vi "Take Composite Image.vi"(7 "Quality":enum16{"perfect", "medium", "low"}(ring), 8 "error in":errorcluster, 9 "Image Name":string="composite image", 10 "Points":refnum<class "Vec3d Class.lvclass">[](array[class]), 11 "CameraTool in":refnum<class "CameraTool Class.lvclass">) -> (0 "error out":errorcluster, 2 "Physical Image":T1, 3 "CameraTool out":refnum<class "CameraTool Class.lvclass">)   [LabVIEW 2011, in "CameraTool Class.lvclass"]
uses:
  CameraTool Class.lvclass
  Vec3d Class/Vec3d Class.lvclass
  Utils/Type Definitions/Physical Image.ctl
  <vilib>/vision/Image Controls.llb/IMAQ Image.ctl
  Config Manager Class/Type Definitions/Camera Enum.ctl
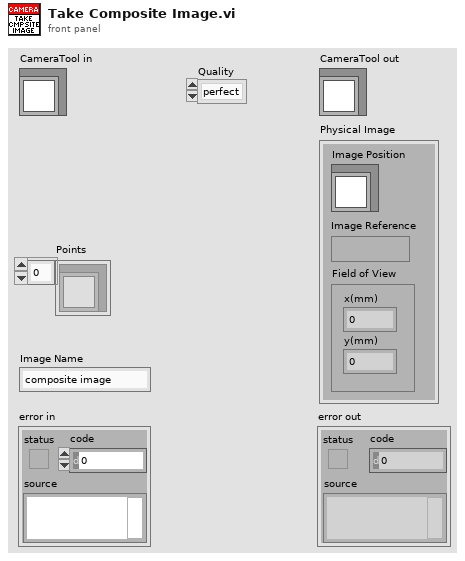
[diagram p1: front panel]
types:
  T1 = typedef "Physical Image.ctl" = cluster{"Image Position":refnum<class "Vec3d Class.lvclass">, "Image Reference":T2, "Field of View":cluster{"x(mm)":dbl, "y(mm)":dbl}}
  T2 = typedef "IMAQ Image.ctl" = refnum<image>
  T3 = typedef "Camera Enum.ctl" = enum16{"GANTRY HEAD", "NEEDLE CALIBRATION X", "NEEDLE CALIBRATION Y"}
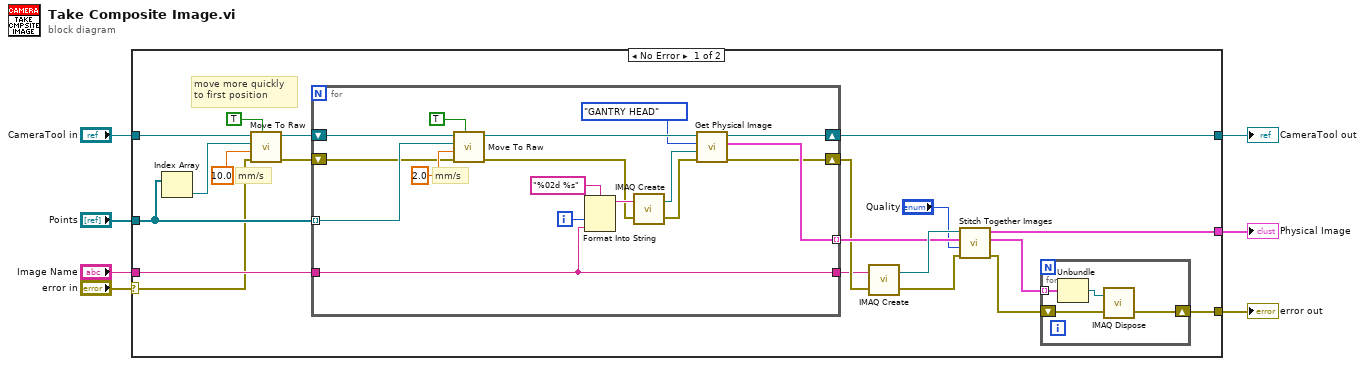
[diagram p0: block diagram]
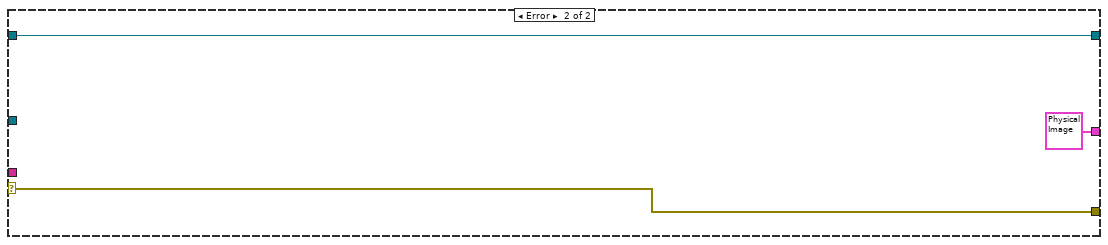
[diagram p2: hidden frame]
diagram:
  n1 = case shown="No Error" "error in" {
    selector: "error in" -> [w9 w51]
    tunnel: [w16 w51] -> w6
    tunnel: [w27 w50] -> w4
    tunnel: "CameraTool in" -> [w13 w50]
    tunnel: "Points" -> [w12 _]
    tunnel: "Image Name" -> [w23 _]
    tunnel: [w19 T1 {"Image Position"=refnum, "Image Reference"=refnum, "Field of View"={"x(mm)"=0.0, "y(mm)"=0.0}} ("Composite Physical Image")] -> w1
    frame No Error {
      # "move more quickly\nto first position"
      # "mm/s"
      n2 = Index Array(array=w12) -> (element=w11:refnum<class "Vec3d Class.lvclass">)  [unwired: 1 in]
      n3 = call-dynamic "Move To Raw.vi"("Wait?"=TRUE, "error in"=w9, "Speed"=10.0, "Destination"=w11, "Gantry in"=w13) -> ("error out"=w8:errorcluster, "Gantry out"=w10:refnum<class "CameraTool Class.lvclass">)  [unwired: 5 in]
      n4 = for {
        shift-right: [w35] -> w24
        shift-left: w8 -> [w36]
        shift-right: [w46] -> w27
        shift-left: w10 -> [w48]
        tunnel: w12 -> [w44] mode=indexing
        tunnel: [w37] -> w25 mode=indexing
        tunnel: [w34] -> w22
        tunnel: w23 -> [w34]
        i -> [w33]
        # "mm/s"
        n5 = call-dynamic "Move To Raw.vi"("Wait?"=TRUE, "error in"=w36, "Speed"=2.0, "Destination"=w44, "Gantry in"=w48) -> ("error out"=w40:errorcluster, "Gantry out"=w47:refnum<class "CameraTool Class.lvclass">)  [unwired: 5 in]
        n6 = Format Into String(format string="%02d %s", w33, w34) -> (resulting string=w41:string)  [unwired: 2 in, 1 out]
        n7 = call "IMAQ Create"("Image Name"=w41, "error in (no error)"=w40) -> ("New Image"=w38:T2, "error out"=w39:errorcluster)  [unwired: 3 in]
        n8 = call-dynamic "Get Physical Image.vi"("error in"=w39, "Image In"=w38, "Camera Name"=Camera_Enum."GANTRY HEAD", "Gantry in"=w47) -> ("error out"=w35:errorcluster, "Physical Image"=w37:T1, "Gantry out"=w46:refnum<class "CameraTool Class.lvclass">)  [unwired: 5 in]
      }
      n9 = call "IMAQ Create"("Image Name"=w22, "error in (no error)"=w24) -> ("New Image"=w26:T2, "error out"=w21:errorcluster)  [unwired: 3 in]
      n10 = call "Stitch Together Images.vi"("error in"=w21, "Quality"="Quality", "Physical Images in"=w25, "Image Dst"=w26) -> ("error out"=w17:errorcluster, "Physical Images out"=w18:T1[], "Composite Physical Image"=w19:T1)  [unwired: 5 in]
      n11 = for {
        tunnel: w18 -> [w31] mode=indexing
        shift-right: [w28] -> w16
        shift-left: w17 -> [w29]
        n12 = Unbundle(w31) -> ("Image Reference"=w30:T2)  [unwired: 2 out]
        n13 = call "IMAQ Dispose"("Image"=w30, "error in (no error)"=w29) -> ("error out"=w28:errorcluster)  [unwired: 4 in]
      }
    }
    frame Error {
    }
  }
  "error out" <- w6
  "CameraTool out" <- w4
  "Physical Image" <- w1
